vi "Panel.vi"(11 "ColorArrayPanel in":refnum<class "ColorArrayPanel.lvclass">) -> ()   [LabVIEW 2020, in "Nested.lvlib" / "ColorArrayPanel.lvclass"]
uses:
  ColorArrayPanel.lvclass
  OOPanel/Panel/Basic UI State.ctl
  OOPanel/Panel/Panel.lvclass
  OOPanel/OOPanel.lvlib
panel:
  in  "Color Box":u32(colorbox)
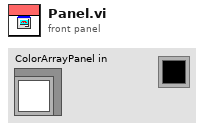
[diagram p1: front panel]
types:
  T1 = typedef "OOPanel.lvlib/Panel.lvclass/Basic UI State.ctl" = enum16{"Init", "Run", "Close"}
  T2 = typedef "OOPanel.lvlib/Panel.lvclass/Panel Events.ctl" = cluster{"Visbility":refnum<user-event>, "Close":refnum<user-event>}
  T3 = typedef "OOPanel.lvlib/Visibility State.ctl" = enum16{"Idle", "Closed", "Hidden", "Visible", "Subpanel", "Hidden Subpanel"}
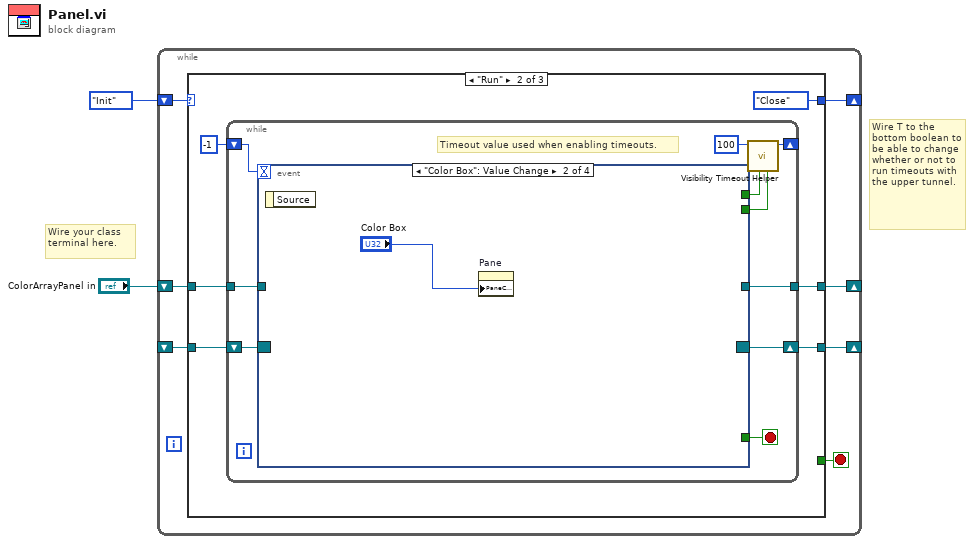
[diagram p0: block diagram]
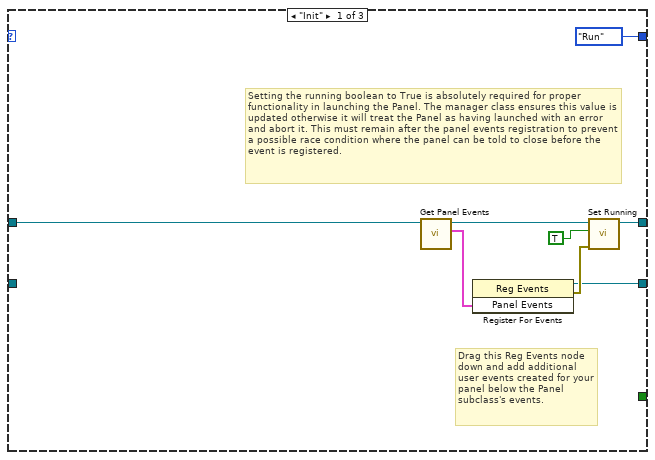
[diagram p2: hidden frame]
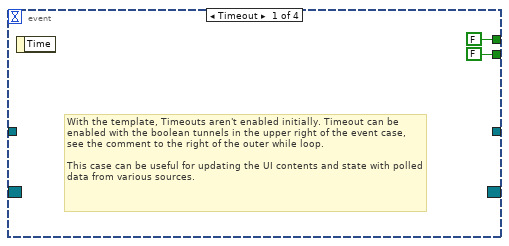
[diagram p3: hidden frame]
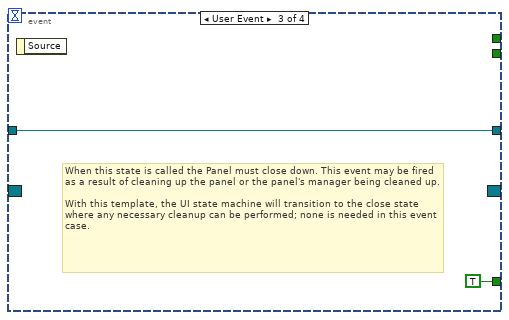
[diagram p4: hidden frame]
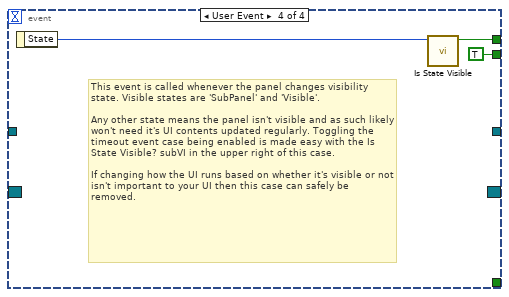
[diagram p5: hidden frame]
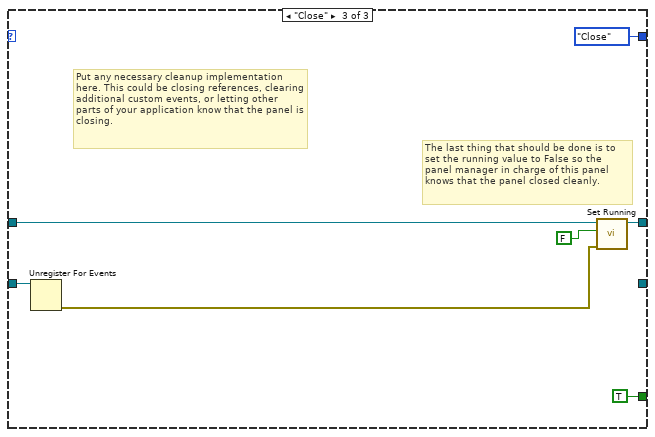
[diagram p6: hidden frame]
diagram:
  # "Wire T to the bottom boolean to be able to change whether or not to run timeouts with the upper tunnel."
  # "Wire your class terminal here."
  n1 = while {
    shift-right: [w8] -> _
    shift-left: _ -> [w9]
    shift-right: [w6] -> _
    shift-left: Basic_UI_State."Init" ("Basic UI State") -> [w7]
    shift-right: [w4] -> _
    shift-left: "ColorArrayPanel in" -> [w3]
    stop <- w5 stop-if-true
    n2 = case shown="\"Run\"" w7 {
      tunnel: w9 -> [_ w23 w44]
      tunnel: [w14 w21 _] -> w8
      tunnel: [Basic_UI_State."Run" ("Basic UI State") Basic_UI_State."Close" ("Basic UI State") Basic_UI_State."Close" ("Basic UI State")] -> w6
      tunnel: [_ _ TRUE] -> w5
      tunnel: [w13 w18 w42] -> w4
      tunnel: w3 -> [w12 w19 w43]
      frame "Init" {
        # "Setting the running boolean to True is absolutely required for proper functionality in launching the Panel. The manager class ensures this value is updated otherwise it will treat the Panel as having launched with an error and abort it. This must remain after the panel events registration to prevent a possible race condition where the panel can be told to close before the event is registered."
        # "Drag this Reg Events node down and add additional user events created for your panel below the Panel subclass's events."
        n3 = call "Get Panel Events.vi"("Panel in"=w12) -> ("Panel Events"=w10:T2, "Panel out"=w11:refnum<class "ColorArrayPanel.lvclass">)  [unwired: 8 in, 1 out]
        n4 = register-events(w10) -> (reference out=w14:refnum<event-registration>, error out=w16:errorcluster)  [unwired: 2 in]
        n5 = call "Set Running.vi"("error in (no error)"=w16, "Running"=TRUE, "Panel in"=w11) -> ("Panel out"=w13:refnum<class "ColorArrayPanel.lvclass">)  [unwired: 7 in, 1 out]
      }
      frame "Run" {
        n6 = while {
          shift-right: [w29] -> w21
          shift-left: w23 -> [w30]
          shift-right: [w32] -> _
          shift-left: -1 ("Timeout") -> [w31]
          tunnel: w19 -> [w25]
          tunnel: [w24] -> w18
          stop <- w26 stop-if-true
          # "Timeout value used when enabling timeouts."
          n7 = event shown="[1] \"Color Box\": Value Change" {
            selector: w30 -> [_ _ _ _]
            dyn-events: [_ _ _ _] -> w29
            timeout: w31 -> [_ _ _ _]
            tunnel: [FALSE _ _ w40] -> w28
            tunnel: [FALSE _ _ TRUE] -> w27
            tunnel: [_ _ TRUE _] -> w26
            tunnel: w25 -> [_ _ w37 _]
            tunnel: [_ _ w37 _] -> w24
            event Timeout {
              # "With the template, Timeouts aren't enabled initially. Timeout can be enabled with the boolean tunnels in the upper right of the event case, see the comment to the right of the outer while loop.\n\nThis case can be useful for updating the UI contents and state with polled data from various sources."
              n8 = event-data() -> ()  [unwired: 1 in, 1 out]
            }
            event "Color Box": Value Change {
              n9 = event-data() -> ()  [unwired: 1 in, 1 out]
              n10 = property on="Pane" class="Pane"("PaneColor"="Color Box") -> ()  [unwired: 2 in, 2 out]
            }
            event User Event {
              # "When this state is called the Panel must close down. This event may be fired as a result of cleaning up the panel or the panel's manager being cleaned up.\n\nWith this template, the UI state machine will transition to the close state where any necessary cleanup can be performed; none is needed in this event case."
              n11 = event-data() -> ()  [unwired: 1 in, 1 out]
            }
            event User Event {
              # "This event is called whenever the panel changes visibility state. Visible states are 'SubPanel' and 'Visible'.\n\nAny other state means the panel isn't visible and as such likely won't need it's UI contents updated regularly. Toggling the timeout event case being enabled is made easy with the Is State Visible? subVI in the upper right of this case.\n\nIf changing how the UI runs based on whether it's visible or not isn't important to your UI then this case can safely be removed."
              n12 = event-data() -> ("State"=w41:T3)  [unwired: 1 in]
              n13 = call "Is State Visible.vi"("Visibility"=w41) -> ("Visible"=w40:bool)  [unwired: 10 in]
            }
          }
          n14 = call "Visibility Timeout Helper.vi"("Update?"=w27, "Use Timeout?"=w28, "Visible Timeout mS"=100) -> ("Timeout"=w32:i32)  [unwired: 8 in]
        }
      }
      frame "Close" {
        # "Put any necessary cleanup implementation here. This could be closing references, clearing additional custom events, or letting other parts of your application know that the panel is closing."
        # "The last thing that should be done is to set the running value to False so the panel manager in charge of this panel knows that the panel closed cleanly."
        n15 = Unregister For Events(event registration refnum=w44) -> (error out=w46:errorcluster)  [unwired: 1 in]
        n16 = call "Set Running.vi"("error in (no error)"=w46, "Running"=FALSE, "Panel in"=w43) -> ("Panel out"=w42:refnum<class "ColorArrayPanel.lvclass">)  [unwired: 7 in, 1 out]
      }
    }
  }
